vi "read_ONE_channel_specify_range_VISA.vi"(5 "postDAQ  wait ms":u32=12, 7 "preDAQ  wait ms":u32=25, 8 "error in":T1, 10 "PD Select":u16(ring) items=["PD1", "PD2", "PD3"], 11 "VISA resource in":refnum<visa-resource-name>) -> (0 "error out":T1, 2 "data":dbl, 3 "VISA resource out":refnum<visa-resource-name>)   [LabVIEW 2024]
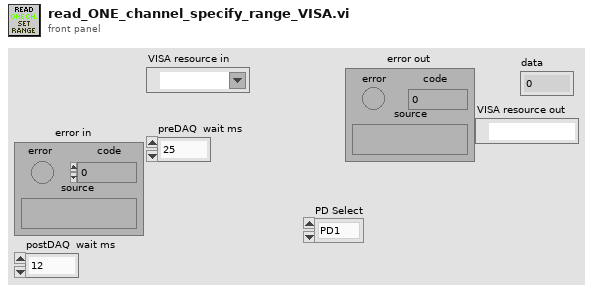
[diagram p1: front panel]
types:
  T1 = cluster{"error":bool, "code":i32, "source":string}
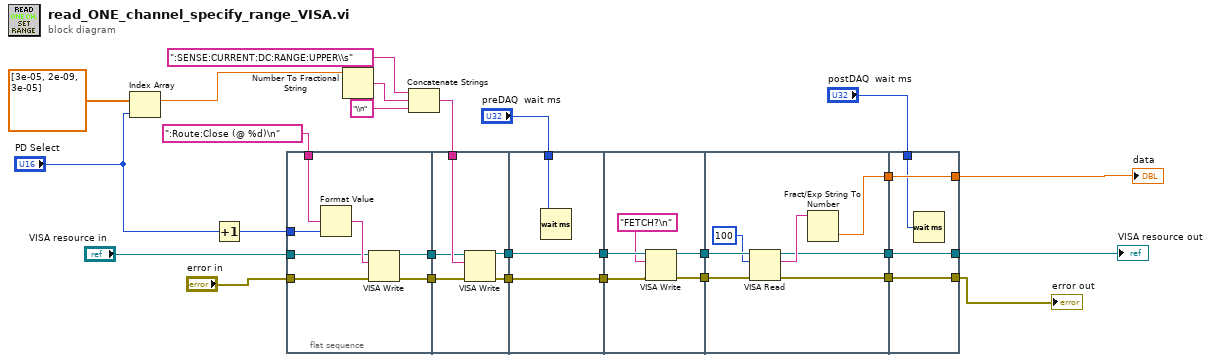
[diagram p0: block diagram]
diagram:
  n1 = Index Array(array=dbl[] [3e-05, 2e-09, 3e-05], index="PD Select") -> (element=w2:dbl)
  n2 = Increment(x="PD Select") -> (x+1=w12:u16)
  n3 = flat-sequence {
    tunnel: w12 -> [w31]
    tunnel: [w32] -> w23
    tunnel: "VISA resource in" -> [w33]
    tunnel: [w30] -> w22
    tunnel: ":Route:Close (@ %d)\n" -> [w29]
    tunnel: "error in" -> [w28]
    tunnel: [w38] -> w21
    tunnel: w23 -> [w39]
    tunnel: w8 -> [w37]
    tunnel: w22 -> [w36]
    tunnel: [w35] -> w20
    tunnel: w21 -> [w42]
    tunnel: [w42] -> w19
    tunnel: "preDAQ  wait ms" -> [w41]
    tunnel: w20 -> [w40]
    tunnel: [w40] -> w18
    tunnel: w19 -> [w47]
    tunnel: w18 -> [w46]
    tunnel: [w44] -> w17
    tunnel: [w43] -> w16
    tunnel: [w50] -> w15
    tunnel: w17 -> [w54]
    tunnel: w16 -> [w53]
    tunnel: [w49] -> w14
    tunnel: [w48] -> w13
    tunnel: [w58] -> w26
    tunnel: w15 -> [w58]
    tunnel: "postDAQ  wait ms" -> [w57]
    tunnel: [w56] -> w24
    tunnel: w14 -> [w56]
    tunnel: [w55] -> w4
    tunnel: w13 -> [w55]
    frame #0 {
      n4 = Format Value(format string=w29, value (0)=w31) -> (output string=w34:string)  [unwired: 1 in]
      n5 = VISA Write(VISA resource name=w33, write buffer=w34, error in (no error)=w28) -> (VISA resource name out=w30:refnum<visa-resource-name>, error out=w32:errorcluster)  [unwired: 1 out]
    }
    frame #1 {
      n6 = VISA Write(VISA resource name=w36, write buffer=w37, error in (no error)=w39) -> (VISA resource name out=w35:refnum<visa-resource-name>, error out=w38:errorcluster)  [unwired: 1 out]
    }
    frame #2 {
      n7 = Wait (ms)(milliseconds to wait=w41) -> ()  [unwired: 1 out]
    }
    frame #3 {
      n8 = VISA Write(VISA resource name=w46, write buffer="FETCH?\n", error in (no error)=w47) -> (VISA resource name out=w44:refnum<visa-resource-name>, error out=w43:errorcluster)  [unwired: 1 out]
    }
    frame #4 {
      n9 = VISA Read(VISA resource name=w54, byte count=u32 100, error in (no error)=w53) -> (VISA resource name out=w49:refnum<visa-resource-name>, read buffer=w51:string, error out=w48:errorcluster)  [unwired: 1 out]
      n10 = Fract/Exp String To Number(string=w51) -> (number=w50:dbl)  [unwired: 3 in, 1 out]
    }
    frame #5 {
      n11 = Wait (ms)(milliseconds to wait=w57) -> ()  [unwired: 1 out]
    }
  }
  n12 = Number To Fractional String(number=w2) -> (F-format string=w11:string)  [unwired: 3 in]
  n13 = Concatenate Strings(":SENSE:CURRENT:DC:RANGE:UPPER\\s", w11, "\\n") -> (w8:string)
  "error out" <- w4
  "data" <- w26
  "VISA resource out" <- w24
